vi "Page_Info_Validate_Filename.vi"(8 "error in (no error)":errorcluster, 10 "Filename in":string, 11 "AB_WebService in":refnum<class "AB_WebService.lvclass">) -> (0 "error out":errorcluster, 1 "hasInvalidCharacters":bool, 2 "Filename out":string, 3 "AB_WebService out":refnum<class "AB_WebService.lvclass">, 5 "message":string)   [LabVIEW 2020, in "AB_WebService.lvclass"]
uses:
  <vilib>/AppBuilder/AB_Classes/WebService/AB_WebService.lvclass
  <resource>/Framework/Providers/Common/provcom_StringGlobals.vi
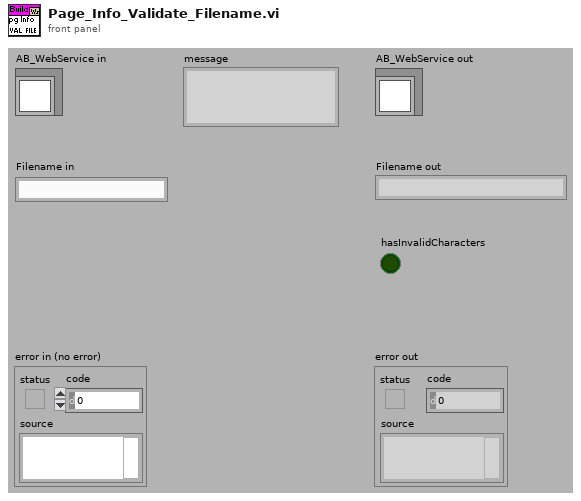
[diagram p1: front panel]
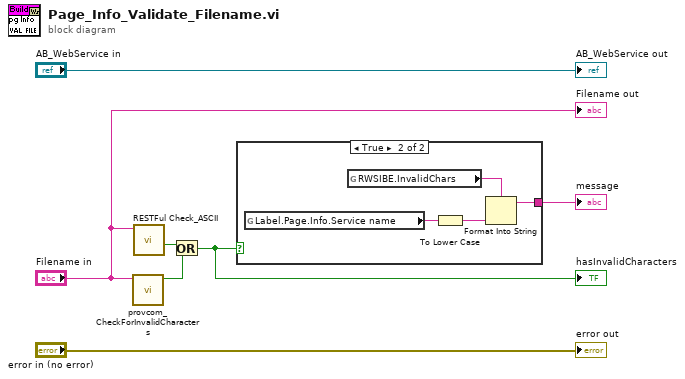
[diagram p0: block diagram]
diagram:
  n1 = call <resource>:"provcom_CheckForInvalidCharacters.vi"("NewString"="Filename in") -> ("HasInvalidCharacters"=w2:bool)  [unwired: 9 in, 1 out]
  n2 = call <vilib>:"RESTFul Check_ASCII.vi"("string in"="Filename in") -> ("invalid chars?"=w3:bool)  [unwired: 9 in, 1 out]
  n3 = Or(x=w3, y=w2) -> (x .or. y?=w1:bool)
  "hasInvalidCharacters" <- w1
  n4 = case shown="True" w1 {
    tunnel: [_ w9] -> w5
    frame False {
    }
    frame True {
      n5 = global read "provcom_StringGlobals.vi" "Label.Page.Info.Service name"() -> (w11:string)
      n6 = global read "provcom_StringGlobals.vi" "RWSIBE.InvalidChars"() -> (w10:string)
      n7 = To Lower Case(string=w11) -> (all lower case string=w8:string)
      n8 = Format Into String(format string=w10, w8) -> (resulting string=w9:string)  [unwired: 2 in, 1 out]
    }
  }
  "message" <- w5
  "error out" <- "error in (no error)"
  "AB_WebService out" <- "AB_WebService in"
  "Filename out" <- "Filename in"
